vi "Test Second Colorv1.vi"(0 "Image":T1, 1 "Mask Image":T1, 3 "Color Ranges":T2) -> (6 "Pixel Area":dbl, 7 "Image Dst Out":T1)   [LabVIEW 2013]
uses:
  <vilib>/vision/Image Controls.llb/IMAQ Image.ctl
  <vilib>/vision/NI_Vision_Development_Module.lvlib
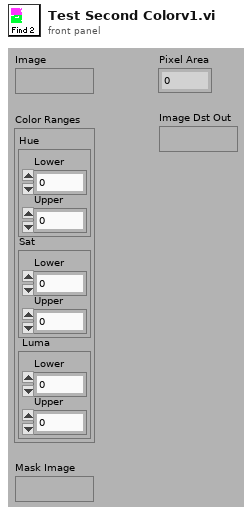
[diagram p1: front panel]
types:
  T1 = typedef "IMAQ Image.ctl" = refnum<image>
  T2 = cluster{"Hue":cluster{"Lower":i32, "Upper":i32}, "Sat":cluster{"Lower":i32, "Upper":i32}, " Luma":cluster{"Lower":i32, "Upper":i32}}
  T3 = cluster{"Pixel Area":dbl, "Rectangle":cluster{"Left":i32, "Top":i32, "Right":i32, "Bottom":i32}, "Additional Measurements":dbl[]}[]
  T4 = cluster{"Pixel Area":dbl, "Rectangle":cluster{"Left":i32, "Top":i32, "Right":i32, "Bottom":i32}, "Additional Measurements":dbl[]}
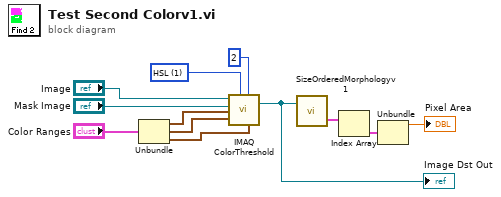
[diagram p0: block diagram]
diagram:
  w5 = u16 1 items=["RGB", "HSL", "HSV", "HSI"] ("Color Mode")
  n1 = Unbundle("Color Ranges") -> ("Hue"=w3:cluster{"Lower":i32, "Upper":i32}, "Sat"=w4:cluster{"Lower":i32, "Upper":i32}, "Luma"=w9:cluster{"Lower":i32, "Upper":i32})
  n2 = call "IMAQ ColorThreshold"("Blue or Luma or Val or Inten Range"=w9, "Replace Value"=2, "Green or Sat Range"=w4, "Color Mode"=w5, "Red or Hue Range"=w3, "Image Dst"="Mask Image", "Image Src"="Image") -> ("Image Dst Out"=w10:T1)  [unwired: 1 in, 3 out]
  "Image Dst Out" <- w10
  n3 = call "SizeOrderedMorphologyv1.vi"("Image Dst Out"=w10) -> ("Particles"=w6:T3)  [unwired: 1 in, 1 out]
  n4 = Index Array(array=w6) -> (element=w7:T4)  [unwired: 1 in]
  n5 = Unbundle(w7) -> ("Pixel Area"=→"Pixel Area":dbl)  [unwired: 2 out]
